vi "Time series viewer warning window caller.vi"   [LabVIEW 2017]
uses:
  Typedefs/Read Write Enum.ctl
  Globals/gl_Time series viewer globals.vi
types:
  T1 = typedef "Read Write Enum.ctl" = enum16{"Read", "Write"}
  T2 = typedef "Time series viewer refs.ctl" = cluster{"This VI":refnum<vi>, "Image control":refnum<vi>, "AVI Mode ind":refnum<vi>, "Play":refnum<vi>, "Stop":refnum<vi>, "Back":refnum<vi>, "Scrollbar":refnum<vi>, "Video length info":refnum<vi>, "Expected speed values":refnum<vi>, "Intensity":refnum<vi>, "Path":refnum<vi>, "Selection sliders":refnum<vi>, "Speed Graph ref":refnum<vi>, "Frame rate set (fps)":refnum<vi>, "Channel to load":refnum<vi>, "Number of rows to generate":refnum<vi>, "Colour":refnum<vi>}
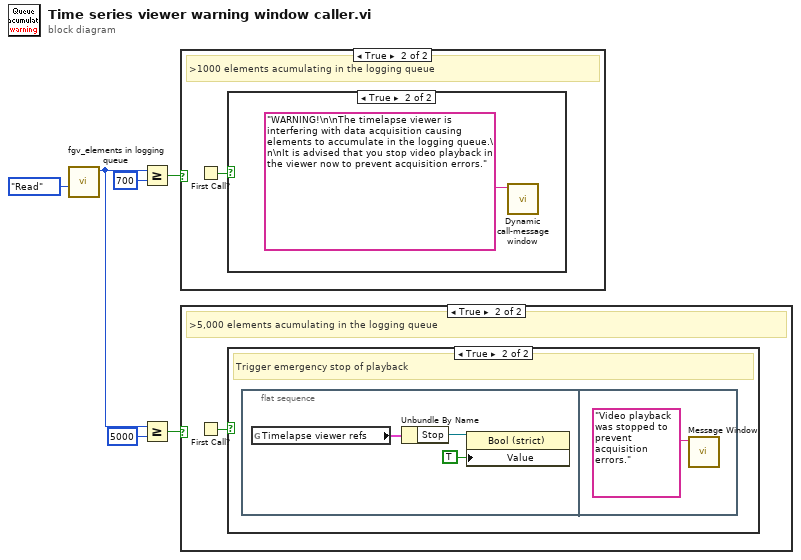
[diagram p0: block diagram]
diagram:
  n1 = call "fgv_elements in logging queue.vi"("Function"=Read_Write_Enum."Read") -> ("Elements in logging queue"=w1:i32)  [unwired: 9 in, 1 out]
  n2 = Greater Or Equal?(x=w1, y=700) -> (x >= y?=w4:bool)
  n3 = Greater Or Equal?(x=w1, y=5000) -> (x >= y?=w3:bool)
  n4 = case shown="True" w4 {
    frame False {
    }
    frame True {
      # ">1000 elements acumulating in the logging queue"
      n5 = First Call?() -> (First Call?: T/F=w7:bool)
      n6 = case shown="True" w7 {
        frame False {
        }
        frame True {
          n7 = call "Dynamic call-message window.vi"("Message"="WARNING!\n\nThe timelapse viewer is interfering with data acquisition causing elements to accumulate in the logging queue.\n\nIt is advised that you stop video playback in the viewer now to prevent acquisition errors." ("Message string")) -> ()  [unwired: 10 in, 1 out]
        }
      }
    }
  }
  n8 = case shown="True" w3 {
    frame False {
    }
    frame True {
      # ">5,000 elements acumulating in the logging queue"
      n9 = First Call?() -> (First Call?: T/F=w9:bool)
      n10 = case shown="True" w9 {
        frame False {
        }
        frame True {
          # "Trigger emergency stop of playback"
          n11 = flat-sequence {
            frame #0 {
              n12 = global read "gl_Time series viewer globals.vi" "Timelapse viewer refs"() -> (w12:T2)
              n13 = Unbundle By Name(w12) -> ("Stop"=w11:refnum<vi>)
              n14 = property class="Bool (strict)"(reference=w11, "Value"=TRUE) -> ()  [unwired: 1 in, 2 out]
            }
            frame #1 {
              n15 = call "Message Window.vi"("Message string"="Video playback was stopped to prevent acquisition errors.") -> ()  [unwired: 10 in, 1 out]
            }
          }
        }
      }
    }
  }
